vi "Get Fields.vi"(8 "error in (no error)":errorcluster, 11 "NMEA Message in":refnum<class "NMEA Message.lvclass">) -> (0 "error out":errorcluster, 2 "Fields":string[](array[string]), 3 "NMEA Message out":refnum<class "NMEA Message.lvclass">)   [LabVIEW 2012, in "nmea.lvlib" / "NMEA Message.lvclass"]
uses:
  NMEA Message.lvclass
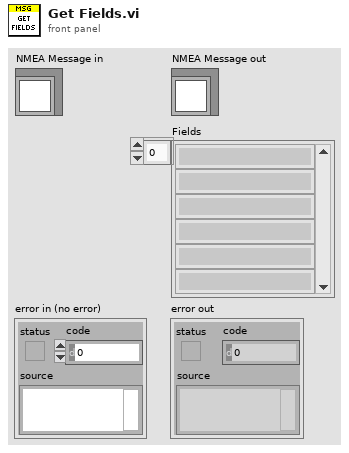
[diagram p1: front panel]
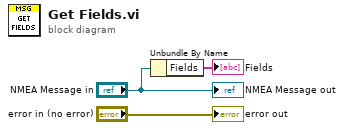
[diagram p0: block diagram]
diagram:
  n1 = Unbundle By Name("NMEA Message in") -> ("Fields"=→"Fields":string[])
  "error out" <- "error in (no error)"
  "NMEA Message out" <- "NMEA Message in"
